vi "Get Object from World.vi"() -> ()   [LabVIEW 2012]
panel:
  out "Time":u32
  out "appended array":dbl[][](array[numeric])
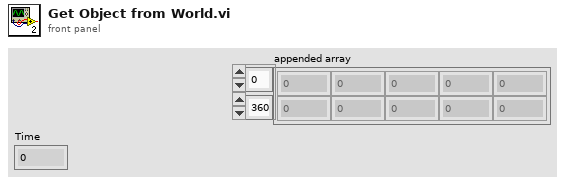
[diagram p1: front panel]
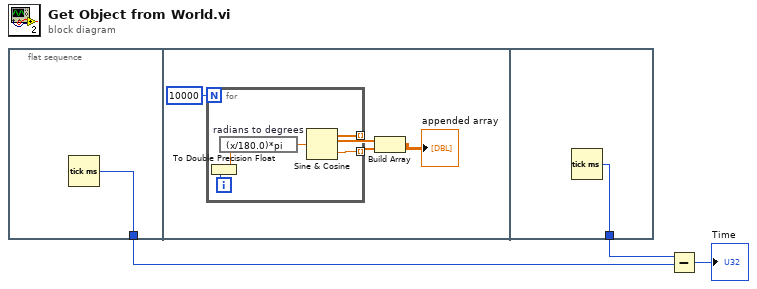
[diagram p0: block diagram]
diagram:
  n1 = flat-sequence {
    tunnel: [w4] -> w3
    tunnel: [w14] -> w2
    frame #0 {
      n2 = Tick Count (ms)() -> (millisecond timer value=w4:u32)
    }
    frame #1 {
      n3 = for {
        N: 10000 -> [_]
        tunnel: [w13] -> w5 mode=indexing
        tunnel: [w12] -> w7 mode=indexing
        i -> [w10]
        n4 = To Double Precision Float(number=w10) -> (double precision float=w9:dbl)
        n5 = expression code="(x/180.0)*pi" "radians to degrees"(w9) -> (w11:dbl)
        n6 = Sine & Cosine(0:w11) -> (1:w13:dbl, 2:w12:dbl)
      }
      n7 = Build Array(w5, w7) -> (→"appended array":dbl[][])
    }
    frame #2 {
      n8 = Tick Count (ms)() -> (millisecond timer value=w14:u32)
    }
  }
  n9 = Subtract(x=w2, y=w3) -> (x-y=→"Time":u32)
